vi "preamp serial write macro.vi"(3 "String":string, 4 "Delay (ms)":i32=250, 5 "VISA resource name":refnum<visa-resource-name>) -> (0 "read buffer":string, 1 "error out":errorcluster, 2 "VISA resource name out":refnum<visa-resource-name>)   [LabVIEW 2014]
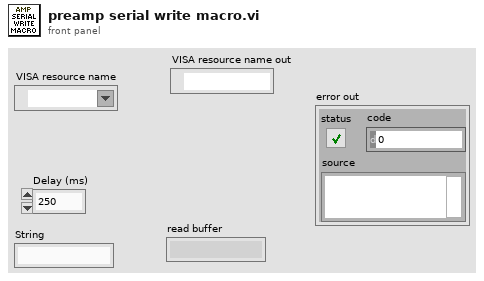
[diagram p1: front panel]
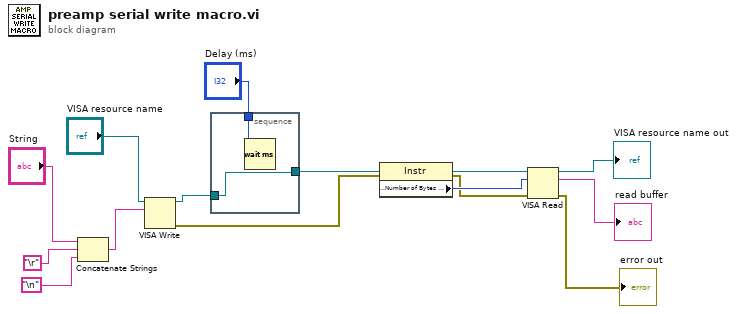
[diagram p0: block diagram]
diagram:
  n1 = Concatenate Strings("String", "\r", "\n") -> (w4:string)
  n2 = VISA Write(VISA resource name="VISA resource name", write buffer=w4) -> (VISA resource name out=w11:refnum<visa-resource-name>, error out=w10:errorcluster)  [unwired: 1 in, 1 out]
  n3 = stacked-sequence {
    tunnel: [w17] -> w15
    tunnel: w11 -> [w17]
    tunnel: "Delay (ms)" -> [w16]
    frame #0 {
      n4 = Wait (ms)(milliseconds to wait=w16) -> ()  [unwired: 1 out]
    }
  }
  n5 = property class="Instr"(reference=w15, error in=w10) -> (reference out=w14:refnum<visa-resource-name>, error out=w12:errorcluster, "Serial Settings:Number of Bytes at Serial Port"=w13:u32)
  n6 = VISA Read(VISA resource name=w14, byte count=w13, error in (no error)=w12) -> (VISA resource name out=→"VISA resource name out":refnum<visa-resource-name>, read buffer=→"read buffer":string, error out=→"error out":errorcluster)  [unwired: 1 out]
